vi "AB Tutorial Acquire.vi"(10 "Array In":dbl[](array[numeric])) -> (0 "Max":dbl, 1 "Min":dbl, 2 "Array Out":dbl[](array[numeric]), 3 "# points acquired":i32)   [LabVIEW 2019]
doc: "This VI is part of an example program for how to use the Application Builder. For more information about this example program please refer to the top level VI \"AB Tutorial GUI.vi\" or the LabVIEW Help for Application Builder."
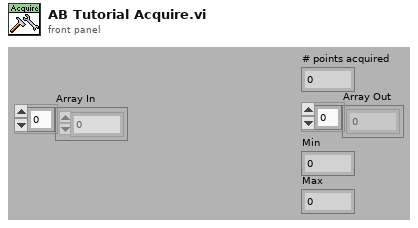
[diagram p1: front panel]
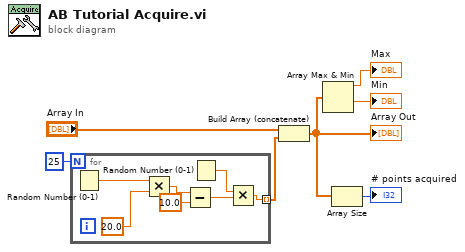
[diagram p0: block diagram]
diagram:
  n1 = for {
    N: 25 -> [_]
    tunnel: [w9] -> w6 mode=indexing
    n2 = Random Number (0-1)() -> (number: 0 to 1=w10:dbl)
    n3 = Multiply(x=w10, y=20.0) -> (x*y=w13:dbl)
    n4 = Subtract(x=w13, y=10.0) -> (x-y=w11:dbl)
    n5 = Random Number (0-1)() -> (number: 0 to 1=w8:dbl)
    n6 = Multiply(x=w8, y=w11) -> (x*y=w9:dbl)
  }
  n7 = Build Array (concatenate)("Array In", w6) -> (w1:dbl[])
  "Array Out" <- w1
  n8 = Array Max & Min(array=w1) -> (max value=→"Max":dbl, min value=→"Min":dbl)  [unwired: 2 out]
  n9 = Array Size(array=w1) -> (size(s)=→"# points acquired":i32)
